vi "Fz_des.vi"() -> ()   [LabVIEW 2018]
panel:
  in  "Fz_des":dbl
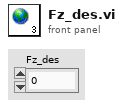
[diagram p1: front panel]
diagram:
